vi "Set Call Chain.vi"(8 "error in (no error)":errorcluster, 10 "Call Chain":string, 11 "Record.Error in":refnum<class "Record.Error.lvclass">) -> (0 "error out":errorcluster, 3 "Record.Error out":refnum<class "Record.Error.lvclass">)   [LabVIEW 2017, in "Error Log.lvlib" / "Record.Error.lvclass"]
uses:
  Record.Error.lvclass
  Record.Error.lvclass/Record.Error.ctl
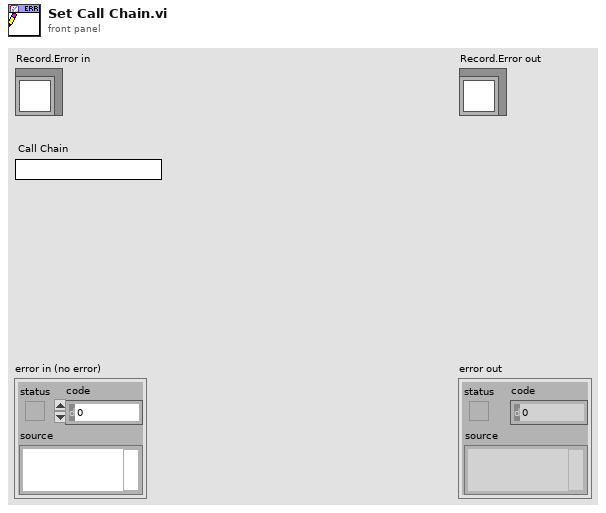
[diagram p1: front panel]
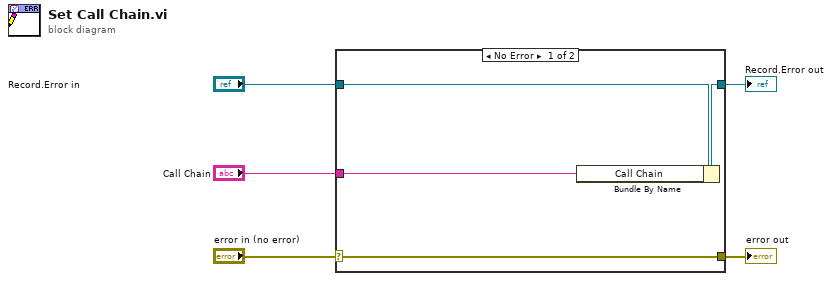
[diagram p0: block diagram]
diagram:
  n1 = case shown="No Error" "error in (no error)" {
    selector: "error in (no error)" -> [w9 w10]
    tunnel: [w9 w10] -> w4
    tunnel: [w7 w11] -> w2
    tunnel: "Record.Error in" -> [w8 w11]
    tunnel: "Call Chain" -> [w6 _]
    frame No Error {
      n2 = Bundle By Name(cluster=w8, "Call Chain"=w6) -> (w7:refnum<class "Record.Error.lvclass">)
    }
    frame Error {
    }
  }
  "error out" <- w4
  "Record.Error out" <- w2
